vi "getDataSize.vi"(6 "Delay between send and receive [ms]":i32=100, 8 "error in (no error)":errorcluster, 11 "CCD in":refnum<class "CCD.lvclass">) -> (0 "error out":errorcluster, 2 "size":i32, 3 "CCD out":refnum<class "CCD.lvclass">)   [LabVIEW 2023, in "CCD.lvclass"]
uses:
  CCD.lvclass
  DataSize.ctl
  20f7d3bd-08ac-4524-9bed-df36c1da25a0.vi
  a21955fc-e3a0-4e36-8495-41f1bfac7860.vi
  <vilib>/JDP Science/JSONtext/Variant to JSON Text.vi
  <vilib>/JDP Science/JSONtext/Set Item.vi
  <vilib>/JDP Science/JSONtext/JSON text to Variant.vi
  <vilib>/JDP Science/JSONtext/LVClass Serializer/JSONtext LVClass Serializer.lvclass
  GenericDevice/GenericDevice.lvclass
  <vilib>/IlluminatedG/lv-web-crypto/lv-json/JSON/JSON.lvlib
panel:
  # "Connector Pane"
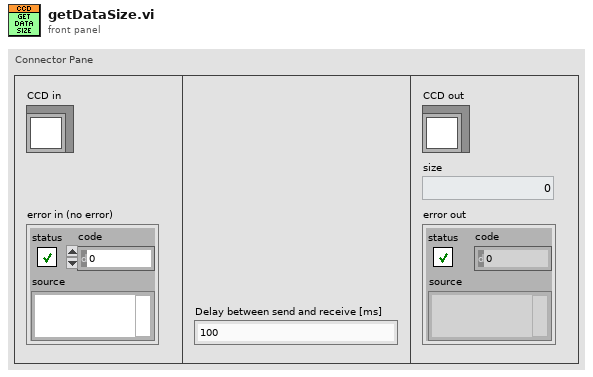
[diagram p1: front panel]
types:
  T1 = typedef "CCD.lvclass/DataSize.ctl" = cluster{"size":i32}
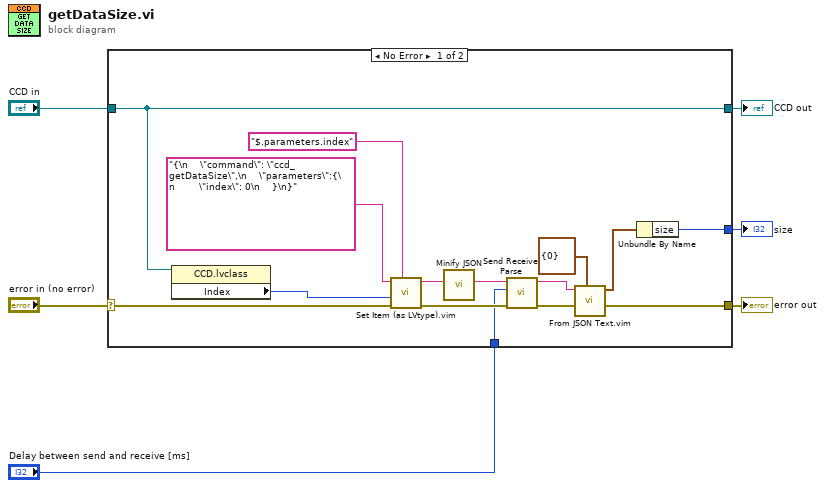
[diagram p0: block diagram]
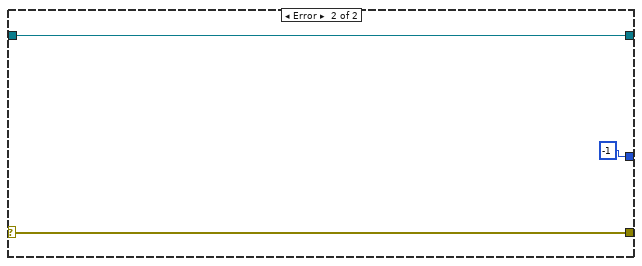
[diagram p2: hidden frame]
diagram:
  n1 = case shown="No Error" "error in (no error)" {
    selector: "error in (no error)" -> [w17 w24]
    tunnel: [w16 w24] -> w5
    tunnel: [w19 w23] -> w3
    tunnel: "CCD in" -> [w19 w23]
    tunnel: [w10 -1 ("size")] -> w2
    tunnel: "Delay between send and receive [ms]" -> [w7 _]
    frame No Error {
      n2 = property class="CCD.lvclass"(reference=w19) -> ("Index"=w18:i32)  [unwired: 1 in, 2 out]
      n3 = call "Set Item (as LVtype).vim"("$Path or Item Name"="$.parameters.index", "error in (no error)"=w17, "Anything"=w18, "JSON"="{\n    \"command\": \"ccd_getDataSize\",\n    \"parameters\":{\n        \"index\": 0\n    }\n}") -> ("error out"=w14:errorcluster, "<JSON>"=w9:string)  [unwired: 4 in, 1 out]
      n4 = call <vilib>:"Minify JSON.vi"("JSON String"=w9) -> ("Minified JSON"=w8:string)  [unwired: 10 in]
      n5 = call "Send Receive Parse.vi"("error in"=w14, "Delay between send and receive [ms]"=w7, "<JSON>"=w8) -> ("error out"=w13:errorcluster, "results-JSON string"=w15:string)  [unwired: 6 in, 1 out]
      n6 = call "From JSON Text.vim"("Data Type and Default Value"=T1 {"size"=0} ("DataSize"), "error in (no error)"=w13, "JSON"=w15) -> ("error out"=w16:errorcluster, "Data out"=w11:T1)  [unwired: 7 in]
      n7 = Unbundle By Name(w11) -> ("size"=w10:i32)
    }
    frame Error {
    }
  }
  "error out" <- w5
  "CCD out" <- w3
  "size" <- w2
